vi "test tools call.vi"(8 "error in (no error)":errorcluster) -> (0 "error out":errorcluster, 3 "body":string)   [LabVIEW 2025, in "MCP Server tests.lvlib"]
uses:
  MCP Server tests.lvlib
  <vilib>/addons/_JKI Toolkits/Caraya/classes/Test/Test.lvclass
  <vilib>/addons/_JKI Toolkits/Caraya/classes/Assert/Assert.lvclass
  <vilib>/JDP Science/JSONtext/JSONtext.lvlib
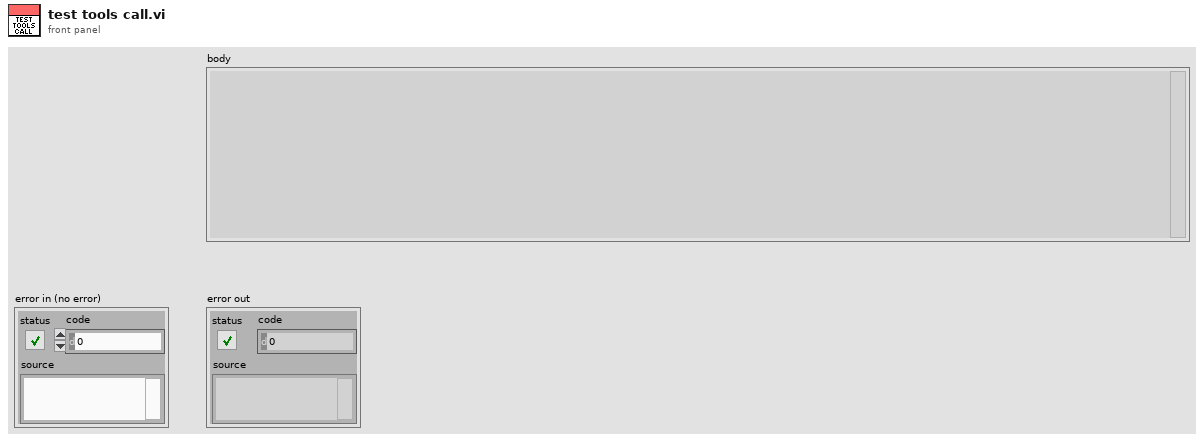
[diagram p1: front panel]
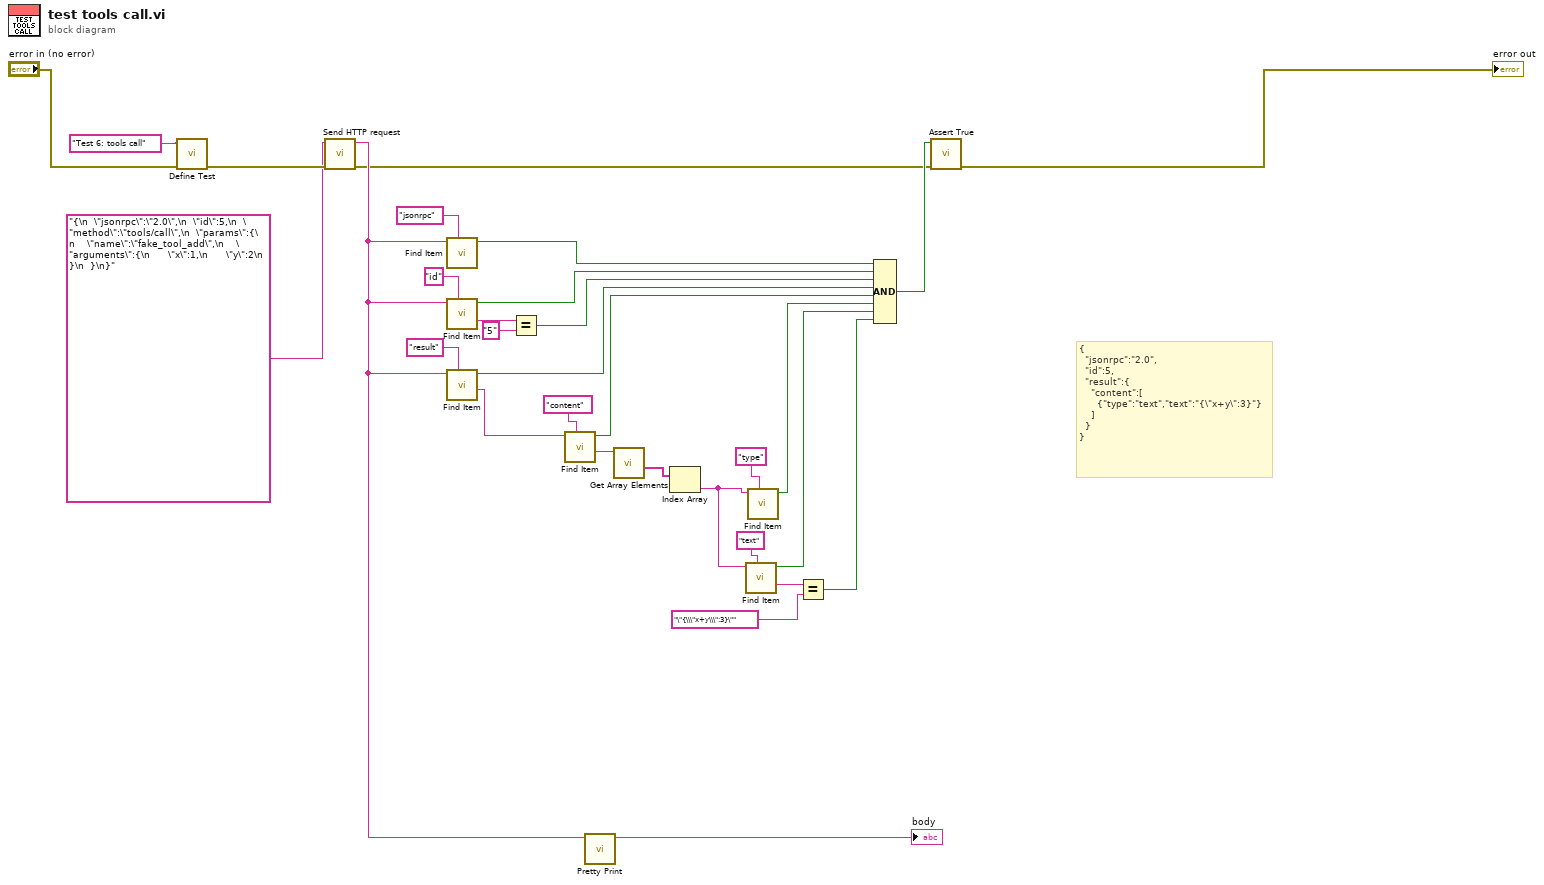
[diagram p0: block diagram]
diagram:
  # "{\n  \"jsonrpc\":\"2.0\",\n  \"id\":5,\n  \"result\":{\n    \"content\":[\n      {\"type\":\"text\",\"text\":\"{\\\"x+y\\\":3}\"}\n    ]\n  }\n}"
  n1 = call <vilib>:"Define Test.vi"("error in (no error)"="error in (no error)", "Label (VI Title)"="Test 6: tools call") -> ("error out"=w18:errorcluster)  [unwired: 8 in, 1 out]
  n2 = call "Send HTTP request.vi"("error in (no error)"=w18, "request"="{\n  \"jsonrpc\":\"2.0\",\n  \"id\":5,\n  \"method\":\"tools/call\",\n  \"params\":{\n    \"name\":\"fake_tool_add\",\n    \"arguments\":{\n      \"x\":1,\n      \"y\":2\n    }\n  }\n}" ("buffer")) -> ("error out"=w19:errorcluster, "response"=w30:string)  [unwired: 8 in]
  n3 = call <vilib>:"Find Item.vi"("$Path or Item Name"="jsonrpc", "JSON"=w30) -> ("Found"=w24:bool)  [unwired: 6 in, 3 out]
  n4 = call <vilib>:"Find Item.vi"("$Path or Item Name"="id", "JSON"=w30) -> ("<JSON>"=w22:string, "Found"=w25:bool)  [unwired: 6 in, 2 out]
  n5 = call <vilib>:"Find Item.vi"("$Path or Item Name"="result", "JSON"=w30) -> ("<JSON>"=w11:string, "Found"=w29:bool)  [unwired: 6 in, 2 out]
  n6 = Equal?(x=w22, y="5") -> (x = y?=w26:bool)
  n7 = call <vilib>:"Find Item.vi"("$Path or Item Name"="content", "JSON"=w11) -> ("<JSON>"=w10:string, "Found"=w12:bool)  [unwired: 6 in, 2 out]
  n8 = call <vilib>:"Pretty Print.vi"("JSON"=w30) -> ("<JSON>"=→"body":string)  [unwired: 8 in, 2 out]
  n9 = call <vilib>:"Get Array Elements.vi"("JSON"=w10) -> ("<JSON>"=w9:string[])  [unwired: 8 in, 2 out]
  n10 = Index Array(array=w9) -> (element=w8:string)  [unwired: 1 in]
  n11 = call <vilib>:"Find Item.vi"("$Path or Item Name"="text", "JSON"=w8) -> ("<JSON>"=w5:string, "Found"=w2:bool)  [unwired: 6 in, 2 out]
  n12 = call <vilib>:"Find Item.vi"("$Path or Item Name"="type", "JSON"=w8) -> ("Found"=w3:bool)  [unwired: 6 in, 3 out]
  n13 = Equal?(x=w5, y="\"{\\\"x+y\\\":3}\"") -> (x = y?=w1:bool)
  n14 = Compound Arithmetic op=AND(w24, w25, w26, w29, w12, w3, w2, w1) -> (w27:bool)
  n15 = call <vilib>:"Assert True.vi"("error in (no error)"=w19, "True?"=w27) -> ("error out"=→"error out":errorcluster)  [unwired: 8 in, 1 out]
